vi "MPM_Set_Trigger_Input_Mode.vi"(8 "error in (no error)":errorcluster, 10 "mode":i32(ring) items=["Internal", "Extarnal"], 11 ".NET Reference in":refnum<k24>) -> (0 "error out":errorcluster, 3 "Reference out":refnum<k24>)   [LabVIEW 2017]
uses:
  LV_IL_Sample/DLL/InstrumentDLL.dll
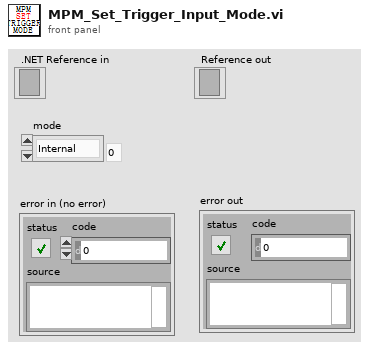
[diagram p1: front panel]
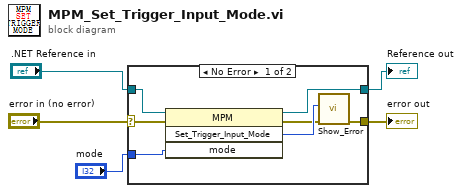
[diagram p0: block diagram]
diagram:
  n1 = case shown="No Error" "error in (no error)" {
    selector: "error in (no error)" -> [w11 w14]
    tunnel: "mode" -> [w12 _]
    tunnel: [w8 w14] -> w3
    tunnel: [w7 w13] -> w2
    tunnel: ".NET Reference in" -> [w6 w13]
    frame No Error {
      n2 = invoke class="MPM" method="Set_Trigger_Input_Mode"(reference=w6, error in=w11, "mode"=w12) -> (reference out=w7:refnum<k24>, error out=w9:errorcluster, "Set_Trigger_Input_Mode"=w10:i32)  [unwired: 1 in, 1 out]
      n3 = call "Show_Error.vi"("error in (no error)"=w9, "Error"=w10) -> ("error out"=w8:errorcluster)  [unwired: 9 in]
    }
    frame Error {
    }
  }
  "Reference out" <- w2
  "error out" <- w3
